vi "Main.vi"(11 "Module Admin":refnum<class "Delacor_lib_QMH_Cloneable Module Admin.lvclass">) -> ()   [LabVIEW 2023, in "TempDataAQuisition.lvlib"]
doc: "This template is based off of the Queued Message Handler design pattern and the Queued Message Handler project template that ships with LabVIEW.\n\nThe main difference is that the queue is private to this module and communication between modules is performed via Broadcast and Request events.\n\nRequest events are wrapped in public API methods and are handled in the Event Handling Loop (EHL) of this VI. Any module can register for Broadcast events sent by this module. The EHL generates messages based on user interface actions.\n\nThe Message Handling Loop (MHL) processes messages generated by the EHL, or by other messages. The messages are string values, so new messages can be added easily to the Message Cases case structure in the MHL. Each message cluster can also provide an optional value for Message Data, which is a variant that can be converted to whatever message-specific data is required.\n_____\nBased on DQMH Project Template 7.0.1.1316."
uses:
  TempDataAQuisition.lvlib
  <vilib>/Delacor/Delacor QMH/Libraries/Cloneable Module Admin_class/Delacor_lib_QMH_Cloneable Module Admin.lvclass
  Module Data--cluster.ctl
  <vilib>/Delacor/Delacor QMH/Libraries/Message Queue_class/Delacor_lib_QMH_Message Queue.lvclass/Delacor_lib_QMH_Message Queue.ctl
  <vilib>/Delacor/Delacor QMH/Libraries/Cloneable Module Admin_class/Delacor_lib_QMH_Cloneable Module Admin.lvclass/Delacor_lib_QMH_Cloneable Module Admin.ctl
  Stop Argument--cluster.ctl
  <vilib>/Delacor/Delacor QMH/Libraries/Module Admin_class/Delacor_lib_QMH_Module Admin.lvclass/Delacor_lib_QMH_Module Admin.ctl
  <vilib>/Utility/miscctls.llb/LVPointTypeDef.ctl
  <vilib>/Delacor/Delacor QMH/Libraries/Message Queue_class/Delacor_lib_QMH_Enqueue Message (Single).vi
  <vilib>/Delacor/Delacor QMH/Libraries/Cloneable Module Admin_class/Delacor_lib_QMH_Get Module ID.vi
  <vilib>/Delacor/Delacor QMH/Libraries/Module Admin_class/Delacor_lib_QMH_Get External Launch.vi
  <vilib>/Delacor/Delacor QMH/Libraries/Message Queue_class/Delacor_lib_QMH_Message Queue.lvclass
  tempRead Argument--cluster.ctl
panel:
  out "error out":errorcluster
  out "Status":string
  in  "Simulate EHL Error":bool
  in  "Simulate MHL Error":bool
  # "Other processes communicate with this Module via its Public API (wrappers for its Request Events).\n\nThis Module communicates with other processes via its Broadcast Events.\nAny process that wants to receive these messages can register for this module's Broadcast events."
  # "This template is for the DQMH framework. See the block diagram for more information on how to use this template."
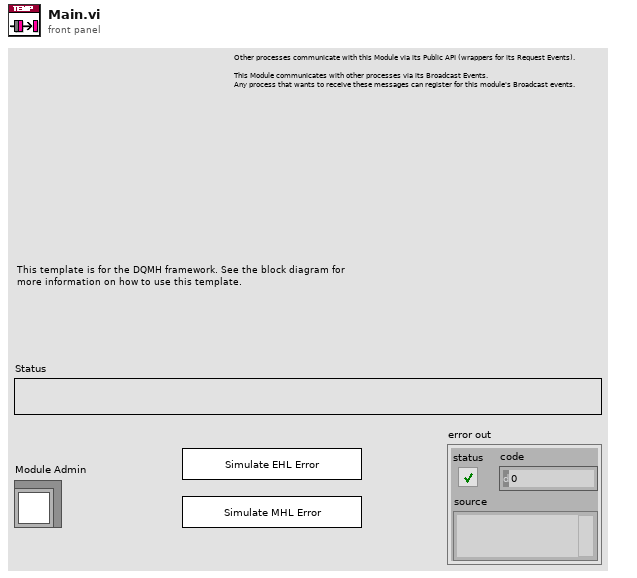
[diagram p1: front panel]
types:
  T1 = typedef "TempDataAQuisition.lvlib/Request Events--cluster.ctl" = cluster{"Stop Module":refnum<user-event>, "Show Panel":refnum<user-event>, "Hide Panel":refnum<user-event>, "Show Diagram":refnum<user-event>, "Get Module Execution Status":refnum<user-event>, "tempRead":refnum<user-event>}
  T2 = typedef "TempDataAQuisition.lvlib/Module Data--cluster.ctl" = cluster{"Status":string}
  T3 = enum32{"invalid lock state", "Not Locked", "Locked (No Password)", "Password-protected"}
  T4 = typedef "TempDataAQuisition.lvlib/Stop Argument--cluster.ctl" = cluster{"Module ID":i32, "Origin":string, "Exit via Stop Module Req?":bool, "Wait for Module to stop?":bool}
  T5 = typedef "TempDataAQuisition.lvlib/tempRead Argument--cluster.ctl" = cluster{"Module ID":i32, "불리언":bool}
  T6 = typedef "LVPointTypeDef.ctl" = cluster{"Horizontal":i16, "Vertical":i16}
  T7 = enum32{"Invalid", "Standard", "Closed", "Hidden", "Minimized", "Maximized"}
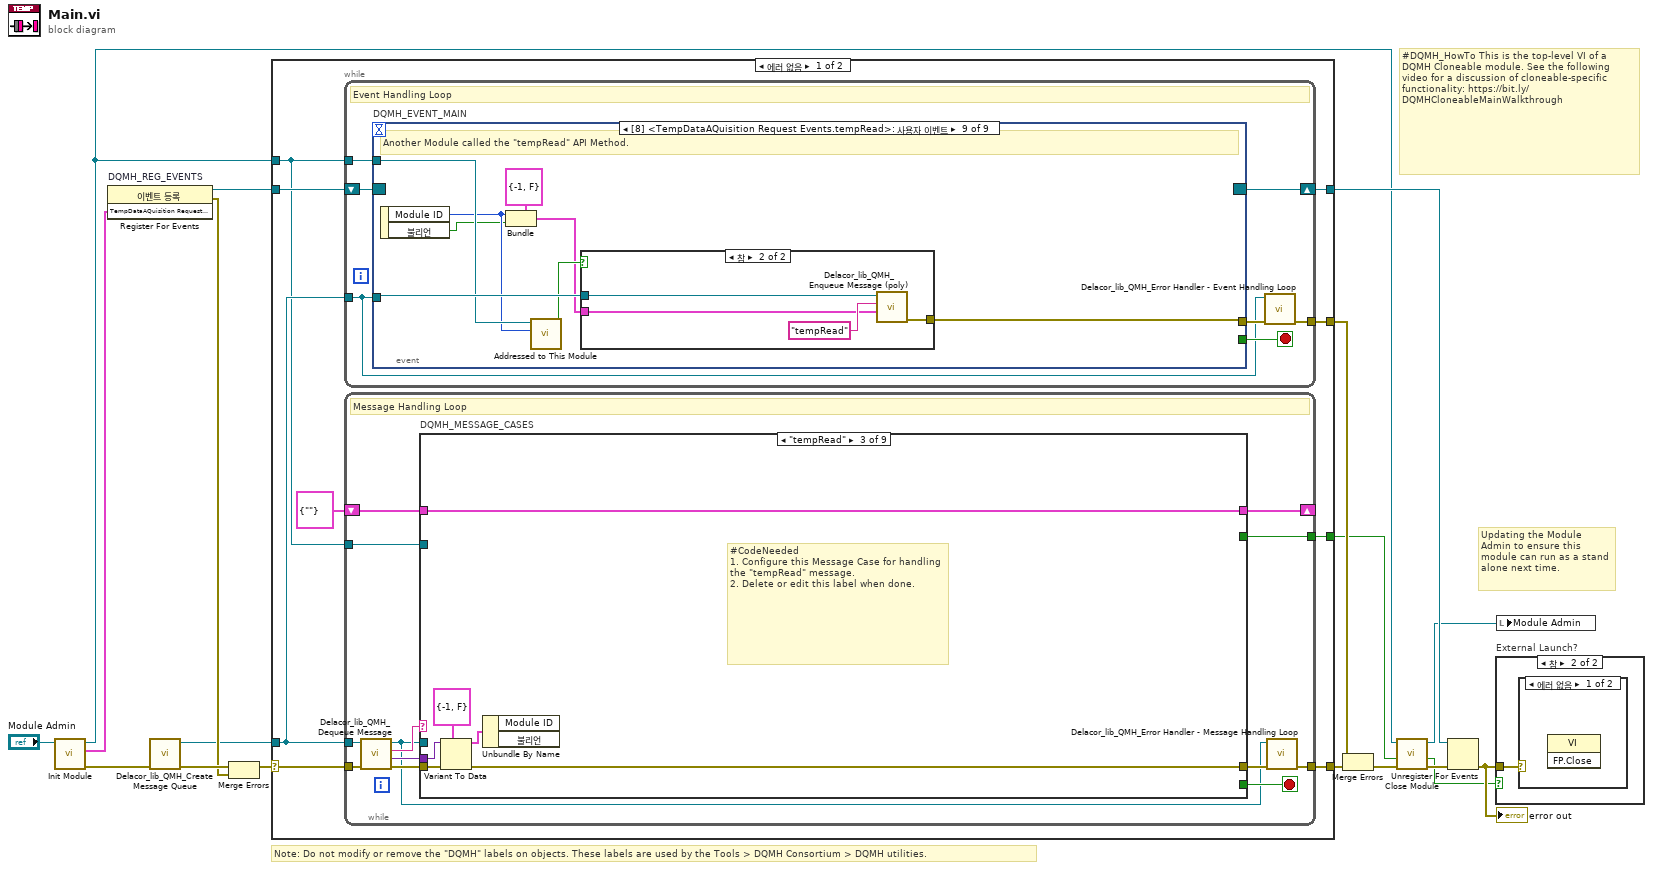
[diagram p0: block diagram]
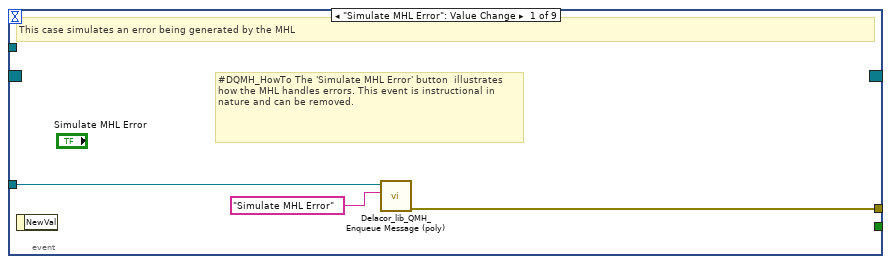
[diagram p2: hidden frame]
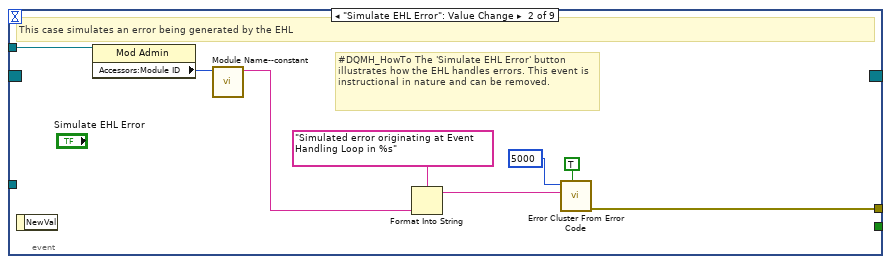
[diagram p3: hidden frame]
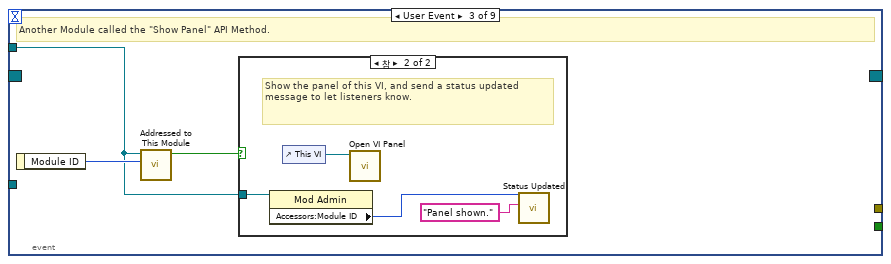
[diagram p4: hidden frame]
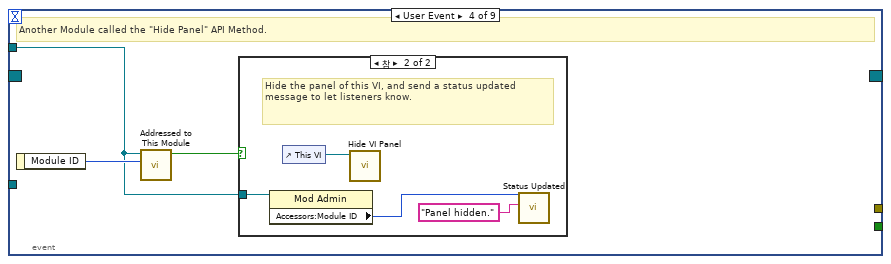
[diagram p6: hidden frame]
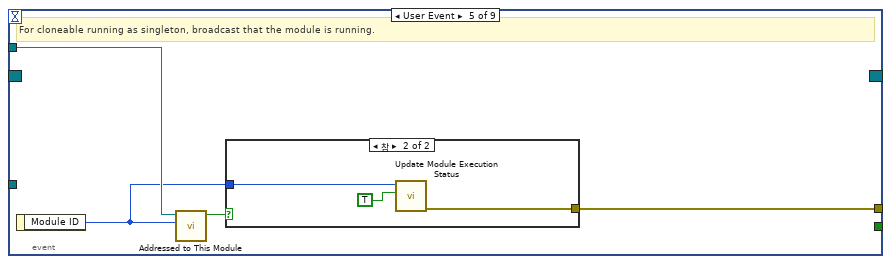
[diagram p8: hidden frame]
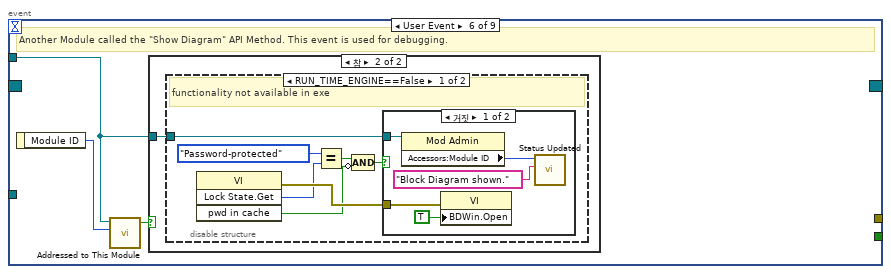
[diagram p10: hidden frame]
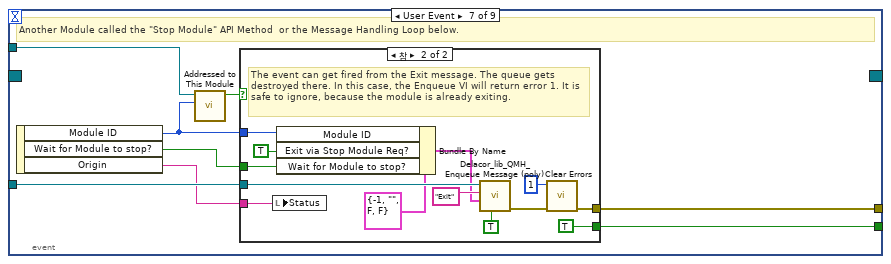
[diagram p14: hidden frame]
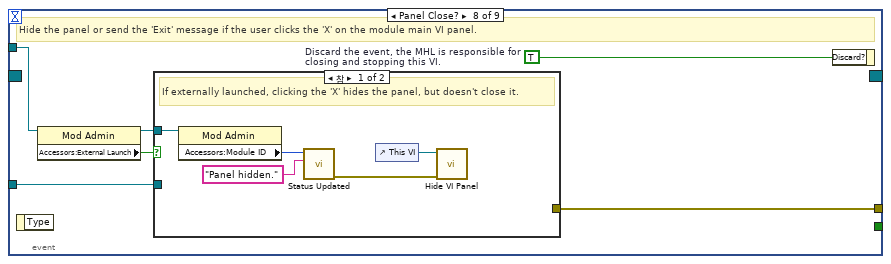
[diagram p16: hidden frame]
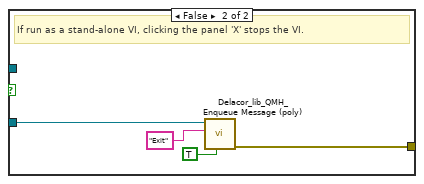
[diagram p17: hidden frame]
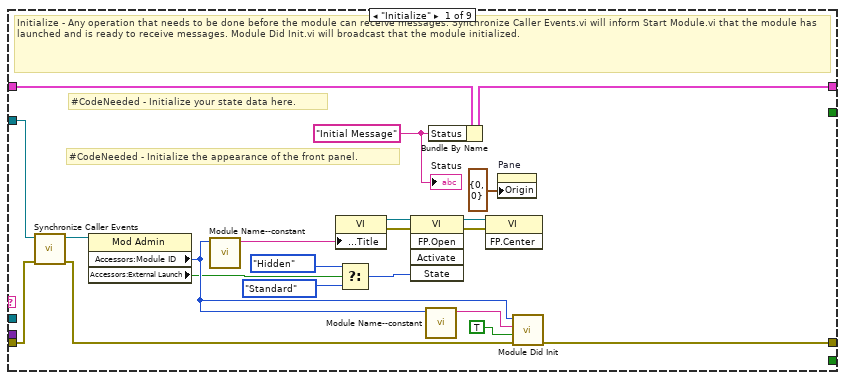
[diagram p19: hidden frame]
diagram:
  # "#DQMH_HowTo This is the top-level VI of a DQMH Cloneable module. See the following video for a discussion of cloneable-specific functionality: https://bit.ly/DQMHCloneableMainWalkthrough"
  # "Note: Do not modify or remove the \"DQMH\" labels on objects. These labels are used by the Tools > DQMH Consortium > DQMH utilities."
  # "Updating the Module Admin to ensure this module can run as a stand alone next time."
  n1 = call "Init Module.vi"("Cloneable Module Admin in"="Module Admin") -> ("error out"=w15:errorcluster, "TempDataAQuisition Request Events"=w7:T1, "Cloneable Module Admin out"=w4:refnum<class "Delacor_lib_QMH_Cloneable Module Admin.lvclass">)  [unwired: 8 in]
  n2 = register-events "DQMH_REG_EVENTS"(w7) -> (reference out=w8:refnum<event-registration>, error out=w10:errorcluster)  [unwired: 2 in]
  n3 = call <vilib>:"Delacor_lib_QMH_Create Message Queue.vi"("error in"=w15) -> ("error out"=w12:errorcluster, "Message Queue"=w6:refnum<class "Delacor_lib_QMH_Message Queue.lvclass">)  [unwired: 9 in]
  n4 = Merge Errors(w12, w10) -> (w11:errorcluster)
  n5 = case shown="에러 없음" w11 {
    selector: w11 -> [w25 w245]
    tunnel: [w27 w244] -> w16
    tunnel: [w24 w243] -> w9
    tunnel: w8 -> [w22 w243]
    tunnel: w6 -> [w21 w236]
    tunnel: [w26 _] -> w17
    tunnel: w4 -> [w20 w239]
    tunnel: [w19 _] -> w2
    frame No Error {
      n6 = while {
        tunnel: w21 -> [w28]
        shift-right: [w31] -> w24
        shift-left: w22 -> [w32]
        tunnel: [w33] -> w26
        tunnel: w20 -> [w29]
        stop <- w30 stop-if-true
        # "Event Handling Loop"
        n7 = event "DQMH_EVENT_MAIN" shown="[8] <TempDataAQuisition Request Events.tempRead>: 사용자 이벤트" {
          selector: w32 -> [_ _ _ _ _ _ _ _ _]
          dyn-events: [_ _ _ _ _ _ _ _ _] -> w31
          timeout: _ -> [_ _ _ _ _ _ _ _ _]
          tunnel: [_ _ _ _ _ _ w86 _ _] -> w30
          tunnel: w28 -> [w36 _ _ _ _ _ w89 w106 w126]
          tunnel: [w37 w45 _ _ w63 _ w90 w109 w119] -> w34
          tunnel: w29 -> [_ w44 w46 w53 w61 w67 w88 w107 w124]
          event "Simulate MHL Error": Value Change {
            # "#DQMH_HowTo The 'Simulate MHL Error' button  illustrates how the MHL handles errors. This event is instructional in nature and can be removed."
            # "This case simulates an error being generated by the MHL"
            n8 = event-data() -> ()  [unwired: 1 in, 1 out]
            n9 = call-poly <vilib>:"Delacor_lib_QMH_Enqueue Message (poly).vi"("Message"="Simulate MHL Error", "Message Queue in"=w36) -> ("error out"=w37:errorcluster)  [unwired: 8 in, 1 out]
          }
          event "Simulate EHL Error": Value Change {
            # "#DQMH_HowTo The 'Simulate EHL Error' button  illustrates how the EHL handles errors. This event is instructional in nature and can be removed."
            # "This case simulates an error being generated by the EHL"
            n10 = event-data() -> ()  [unwired: 1 in, 1 out]
            n11 = property on="Property Node" class="Mod Admin"(reference=w44) -> ("Accessors:Module ID"=w43:i32)  [unwired: 1 in, 2 out]
            n12 = call "Module Name--constant.vi"("Module ID"=w43) -> ("Module Name"=w38:string)  [unwired: 10 in]
            n13 = Format Into String(format string="Simulated error originating at Event Handling Loop in %s", w38) -> (resulting string=w41:string)  [unwired: 2 in, 1 out]
            n14 = call <vilib>:"Error Cluster From Error Code.vi"("show call chain? (False)"=TRUE, "error message (\"\")"=w41, "error code (0)"=5000) -> ("error out"=w45:errorcluster)  [unwired: 6 in]
          }
          event User Event {
            # "Another Module called the \"Show Panel\" API Method."
            n15 = event-data() -> ("Module ID"=w47:i32)  [unwired: 1 in]
            n16 = call "Addressed to This Module.vi"("Module ID from Argument"=w47, "Module Admin"=w46) -> ("Addressed to this instance?"=w48:bool)  [unwired: 8 in, 1 out]
            n17 = case shown="참" w48 {
              tunnel: w46 -> [_ w50]
              frame False {
              }
              frame True {
                # "Show the panel of this VI, and send a status updated message to let listeners know."
                n18 = property on="Property Node" class="Mod Admin"(reference=w50) -> ("Accessors:Module ID"=w49:i32)  [unwired: 1 in, 2 out]
                n19 = control-ref of="This VI"() -> (w52:refnum<vi>)
                n20 = call "Open VI Panel.vi"("VI"=w52) -> ()  [unwired: 10 in, 1 out]
                n21 = call "Status Updated.vi"("Status"="Panel shown." ("format string"), "Module ID"=w49) -> ()  [unwired: 9 in, 1 out]
              }
            }
          }
          event User Event {
            # "Another Module called the \"Hide Panel\" API Method."
            n22 = event-data() -> ("Module ID"=w54:i32)  [unwired: 1 in]
            n23 = call "Addressed to This Module.vi"("Module ID from Argument"=w54, "Module Admin"=w53) -> ("Addressed to this instance?"=w55:bool)  [unwired: 8 in, 1 out]
            n24 = case shown="참" w55 {
              tunnel: w53 -> [_ w57]
              frame False {
              }
              frame True {
                # "Hide the panel of this VI, and send a status updated message to let listeners know."
                n25 = property on="Property Node" class="Mod Admin"(reference=w57) -> ("Accessors:Module ID"=w56:i32)  [unwired: 1 in, 2 out]
                n26 = control-ref of="This VI"() -> (w59:refnum<vi>)
                n27 = call "Hide VI Panel.vi"("VI"=w59) -> ()  [unwired: 10 in, 1 out]
                n28 = call "Status Updated.vi"("Status"="Panel hidden." ("format string"), "Module ID"=w56) -> ()  [unwired: 9 in, 1 out]
              }
            }
          }
          event User Event {
            # "For cloneable running as singleton, broadcast that the module is running."
            n29 = event-data() -> ("Module ID"=w60:i32)  [unwired: 1 in]
            n30 = call "Addressed to This Module.vi"("Module ID from Argument"=w60, "Module Admin"=w61) -> ("Addressed to this instance?"=w62:bool)  [unwired: 8 in, 1 out]
            n31 = case shown="참" w62 {
              tunnel: [_ w66] -> w63
              tunnel: w60 -> [_ w65]
              frame False {
              }
              frame True {
                n32 = call "Update Module Execution Status.vi"("Running?"=TRUE, "Module ID"=w65) -> ("error out"=w66:errorcluster)  [unwired: 9 in]
              }
            }
          }
          event User Event {
            # "Another Module called the \"Show Diagram\" API Method. This event is used for debugging."
            n33 = event-data() -> ("Module ID"=w68:i32)  [unwired: 1 in]
            n34 = call "Addressed to This Module.vi"("Module ID from Argument"=w68, "Module Admin"=w67) -> ("Addressed to this instance?"=w69:bool)  [unwired: 8 in, 1 out]
            n35 = case shown="참" w69 {
              tunnel: w67 -> [_ w70]
              frame False {
              }
              frame True {
                n36 = disable-structure shown="RUN_TIME_ENGINE==False" {
                  disable-tunnel: w70 -> [w71 _]
                  frame condition #0 (active) {
                    # "functionality not available in exe"
                    n37 = invoke on="Invoke Node" class="VI" method="Lock State.Get"() -> (error out=w77:errorcluster, "Get Lock State"=w76:T3, "pwd in cache"=w73:bool)  [unwired: 4 in, 1 out]
                    n38 = Equal?(x=T3."Password-protected", y=w76) -> (x = y?=w74:bool)
                    n39 = Compound Arithmetic op=AND(w74, invert w73) -> (w72:bool)
                    n40 = case shown="거짓" w72 {
                      tunnel: w77 -> [w82 _]
                      tunnel: w71 -> [w79 _]
                      frame False {
                        n41 = property on="Property Node" class="Mod Admin"(reference=w79) -> ("Accessors:Module ID"=w78:i32)  [unwired: 1 in, 2 out]
                        n42 = property on="Property Node" class="VI"(error in=w82, "BDWin.Open"=TRUE ("Block Diagram Window:Open")) -> ()  [unwired: 1 in, 2 out]
                        n43 = call "Status Updated.vi"("Status"="Block Diagram shown." ("format string"), "Module ID"=w78) -> ()  [unwired: 9 in, 1 out]
                      }
                      frame True {
                        # "Password-protected VI, and the password is not in the cache. Do not show the diagram."
                      }
                    }
                  }
                  frame condition #1 {
                  }
                }
              }
            }
          }
          event User Event {
            # "Another Module called the \"Stop Module\" API Method  or the Message Handling Loop below."
            n44 = event-data() -> ("Module ID"=w84:i32, "Wait for Module to stop?"=w85:bool, "Origin"=w83:string)  [unwired: 1 in]
            n45 = call "Addressed to This Module.vi"("Module ID from Argument"=w84, "Module Admin"=w88) -> ("Addressed to this instance?"=w87:bool)  [unwired: 8 in, 1 out]
            n46 = case shown="참" w87 {
              tunnel: [_ w102] -> w90
              tunnel: w89 -> [_ w98]
              tunnel: [_ TRUE] -> w86
              tunnel: w85 -> [_ w93]
              tunnel: w84 -> [_ w95]
              tunnel: w83 -> [_ w91]
              frame False {
              }
              frame True {
                # "The event can get fired from the Exit message. The queue gets destroyed there. In this case, the Enqueue VI will return error 1. It is safe to ignore, because the module is already exiting."
                n47 = local write "Status"(w91) -> ()
                n48 = Bundle By Name(cluster=T4 {"Module ID"=-1, "Origin"="", "Exit via Stop Module Req?"=FALSE, "Wait for Module to stop?"=FALSE} ("Stop Argument"), "Module ID"=w95, "Exit via Stop Module Req?"=TRUE, "Wait for Module to stop?"=w93) -> (w92:T4)
                n49 = call-poly <vilib>:"Delacor_lib_QMH_Enqueue Message (poly).vi"("Priority Message? (F)"=TRUE, "Message Data"=w92, "Message"="Exit", "Message Queue in"=w98) -> ("error out"=w103:errorcluster)  [unwired: 6 in, 1 out]
                n50 = call <vilib>:"Clear Errors.vi"("error in (no error)"=w103, "specific error code to clear (0: all)"=1) -> ("error out"=w102:errorcluster)  [unwired: 4 in, 1 out]
              }
            }
          }
          event Panel Close? {
            w108 = TRUE  # Discard the event, the MHL is responsible for closing and stopping this VI.
            # "Hide the panel or send the 'Exit' message if the user clicks the 'X' on the module main VI panel."
            n51 = event-data() -> ()  [unwired: 1 in, 1 out]
            n52 = property on="Property Node" class="Mod Admin"(reference=w107) -> (reference out=w104:refnum<class "Delacor_lib_QMH_Cloneable Module Admin.lvclass">, "Accessors:External Launch"=w105:bool)  [unwired: 1 in, 1 out]
            n53 = case shown="참" w105 {
              tunnel: w106 -> [_ w117]
              tunnel: [_ w118] -> w109
              tunnel: w104 -> [w112 _]
              frame True {
                # "If externally launched, clicking the 'X' hides the panel, but doesn't close it."
                n54 = property on="Property Node" class="Mod Admin"(reference=w112) -> ("Accessors:Module ID"=w111:i32)  [unwired: 1 in, 2 out]
                n55 = call "Status Updated.vi"("Status"="Panel hidden." ("format string"), "Module ID"=w111) -> ("error out"=w110:errorcluster)  [unwired: 9 in]
                n56 = control-ref of="This VI"() -> (w114:refnum<vi>)
                n57 = call "Hide VI Panel.vi"("error in"=w110, "VI"=w114) -> ()  [unwired: 9 in, 1 out]
              }
              frame False {
                # "If run as a stand-alone VI, clicking the panel 'X' stops the VI."
                n58 = call-poly <vilib>:"Delacor_lib_QMH_Enqueue Message (poly).vi"("Priority Message? (F)"=TRUE, "Message"="Exit", "Message Queue in"=w117) -> ("error out"=w118:errorcluster)  [unwired: 7 in, 1 out]
              }
            }
            n59 = event-data ("Event Filter Node")("Discard?"=w108) -> ()  [unwired: 1 in, 1 out]
          }
          event User Event {
            # "Another Module called the \"tempRead\" API Method."
            n60 = event-data() -> ("Module ID"=w121:i32, "불리언"=w120:bool)  [unwired: 1 in]
            n61 = Bundle(cluster=T5 {"Module ID"=-1, "불리언"=FALSE} ("tempRead Argument"), "Module ID"=w121, "불리언"=w120) -> (w122:T5)
            n62 = call "Addressed to This Module.vi"("Module ID from Argument"=w121, "Module Admin"=w124) -> ("Addressed to this instance?"=w125:bool)  [unwired: 8 in, 1 out]
            n63 = case "케이스 구조" shown="참" w125 {
              tunnel: w126 -> [_ w130]
              tunnel: w122 -> [_ w128]
              tunnel: [_ w127] -> w119
              frame False {
              }
              frame True {
                n64 = call-poly <vilib>:"Delacor_lib_QMH_Enqueue Message (poly).vi"("Message Data"=w128, "Message"="tempRead", "Message Queue in"=w130) -> ("error out"=w127:errorcluster)  [unwired: 7 in, 1 out]
              }
            }
          }
        }
        n65 = call-dynamic "Delacor_lib_QMH_Error Handler - Event Handling Loop.vi"("error in"=w34, "Message Queue in"=w28) -> ("dup error in"=w33:errorcluster)  [unwired: 8 in, 1 out]
      }
      n66 = while {
        tunnel: w21 -> [w131]
        shift-right: [w138] -> _
        shift-left: T2 {"Status"=""} ("Data Cluster") -> [w139]
        tunnel: w25 -> [w142]
        tunnel: [w140] -> w27
        tunnel: w20 -> [w133]
        tunnel: [w132] -> w19
        stop <- w137 stop-if-true
        # "Message Handling Loop"
        n67 = call-dynamic "Delacor_lib_QMH_Dequeue Message.vi"("error in"=w142, "Message Queue in"=w131) -> ("error out"=w141:errorcluster, "Message Data"=w135:variant, "Message"=w136:string, "Message Queue out"=w134:refnum<class "Delacor_lib_QMH_Message Queue.lvclass">)  [unwired: 6 in]
        n68 = case "DQMH_MESSAGE_CASES" shown="\"tempRead\"" w136 {
          selector: w136 -> [_ _ _ _ _ _ _ _ w225]
          tunnel: w134 -> [_ _ _ _ _ w180 _ w217 _]
          tunnel: w141 -> [w162 w166 w172 w175 w177 w189 w206 w223 w234]
          tunnel: [w160 w166 w170 w174 w177 w185 w205 w218 w235] -> w143
          tunnel: w139 -> [w153 w165 w171 w173 w176 w184 w203 w216 w232]
          tunnel: [w152 w165 w171 w173 w176 w184 w203 w216 w232] -> w138
          tunnel: [_ _ _ _ _ _ _ w215 _] -> w137
          tunnel: w135 -> [_ _ w169 _ _ w183 _ w213 _]
          tunnel: w133 -> [w147 _ _ _ _ w182 w201 w208 w231]
          tunnel: [_ _ _ _ _ _ _ w211 _] -> w132
          frame "Initialize" {
            w144 = "Initial Message" ("Initial Message")
            # "#CodeNeeded - Initialize the appearance of the front panel."
            # "#CodeNeeded - Initialize your state data here."
            # "Initialize - Any operation that needs to be done before the module can receive messages. Synchronize Caller Events.vi will inform Start Module.vi that the module has launched and is ready to receive messages. Module Did Init.vi will broadcast that the module initialized."
            n69 = call "Synchronize Caller Events.vi"("error in"=w162, "Module Admin"=w147) -> ("error out"=w161:errorcluster, "Module Admin out"=w146:refnum<class "Delacor_lib_QMH_Cloneable Module Admin.lvclass">)  [unwired: 8 in]
            n70 = property on="Property Node" class="Mod Admin"(reference=w146) -> ("Accessors:Module ID"=w149:i32, "Accessors:External Launch"=w148:bool)  [unwired: 1 in, 2 out]
            n71 = call "Module Name--constant.vi"("Module ID"=w149) -> ("Module Name"=w157:string)  [unwired: 10 in]
            n72 = property on="Property Node" class="VI"("Front Panel.Title"=w157) -> (reference out=w159:refnum<vi>, error out=w164:errorcluster)  [unwired: 2 in]
            n73 = Select(t=T7."Hidden" ("State"), s=w148, f=T7."Standard" ("State")) -> (s? t:f=w154:T7)
            n74 = invoke on="Invoke Node" class="VI" method="FP.Open"(reference=w159, error in=w164, "State"=w154) -> (reference out=w158:refnum<vi>, error out=w163:errorcluster)  [unwired: 2 in, 3 out]
            n75 = call "Module Name--constant.vi"("Module ID"=w149) -> ("Module Name"=w150:string)  [unwired: 10 in]
            n76 = Bundle By Name(cluster=w153, "Status"=w144) -> (w152:T2)
            n77 = invoke on="Invoke Node" class="VI" method="FP.Center"(reference=w158, error in=w163) -> ()  [unwired: 1 in, 3 out]
            n78 = property on="Pane" class="Pane"("Origin"=T6 {"Horizontal"=0, "Vertical"=0}) -> ()  [unwired: 2 in, 2 out]
            n79 = call "Module Did Init.vi"("error in"=w161, "Initialized?"=TRUE, "Origin"=w150, "Module ID"=w149) -> ("error out"=w160:errorcluster)  [unwired: 7 in]
            "Status" <- w144
          }
          frame "---Module Specific---" {
            # "Separator -- The following cases handle messages specific to this Module."
          }
          frame "tempRead" {
            # "#CodeNeeded\n1. Configure this Message Case for handling the \"tempRead\" message.\n2. Delete or edit this label when done."
            n80 = Variant To Data(error in=w172, type=T5 {"Module ID"=-1, "불리언"=FALSE} ("tempRead Argument"), Variant=w169) -> (data=w167:T5, error out=w170:errorcluster)
            n81 = Unbundle By Name(w167) -> ()  [unwired: 2 out]
          }
          frame "---Copy This Frame---" {
            # "Duplicate this frame when creating new messages.  Change this comment in the duplicated frame to describe this message."
            n82 = Merge Errors(w175) -> (w174:errorcluster)
          }
          frame "---Exit and Error Handling---" {
            # "Separator - the following cases handle errors and exit messages."
          }
          frame "Error" {
            # "#CodeRecommended - If the module is running in standalone mode (External Launch = FALSE), this code will pop up an error dialog and call the 'Exit' message if an error occurs. Add more fine-grained error management here."
            # "Error - Check the error message data and respond accordingly. This message is sent by the \"Error Handler\" VIs at the end of each loop in this application."
            n83 = property on="Property Node" class="Mod Admin"(reference=w182) -> ("Accessors:External Launch"=w181:bool, "Accessors:Module ID"=w179:i32)  [unwired: 1 in, 2 out]
            n84 = Variant To Data(error in=w189, type=errorcluster {"status"=FALSE, "code"=0, "source"=""} ("error constant"), Variant=w183) -> (data=w178:errorcluster, error out=w187:errorcluster)
            n85 = local write "error out"(w178) -> ()
            n86 = call "Error Reported.vi"("Error"=w178, "Module ID"=w179) -> ()  [unwired: 9 in, 1 out]
            n87 = case shown="거짓" w181 {
              tunnel: [w194 _] -> w186
              tunnel: w180 -> [w192 _]
              tunnel: w178 -> [w193 _]
              frame False {
                n88 = disable-structure shown="DQMH_Disable_SEH==TRUE" {
                  disable-tunnel: w193 -> [w195 _]
                  frame condition #0 (active) {
                    # "If the module is running standalone, then pop up an error dialog and call the \"Exit\" message."
                    n89 = call <vilib>:"Simple Error Handler.vi"("error in (no error)"=w195) -> ()  [unwired: 4 in, 5 out]
                  }
                  frame condition #1 {
                    # "To prevent the Simple Error Handler VI from being loaded (e.g. when deploying to a Real-Time target), add the Conditional Disable Symbol \"DQMH_Disable_SEH\" to your project and set it to TRUE."
                  }
                }
                n90 = call-poly <vilib>:"Delacor_lib_QMH_Enqueue Message (poly).vi"("Priority Message? (F)"=TRUE, "Message"="Exit", "Message Queue in"=w192) -> ("error out"=w194:errorcluster)  [unwired: 7 in, 1 out]
              }
              frame True {
                # "If the module was launched externally, calling the Error Reported broadcast VI is the only action performed by the \"Error\" message. The module's caller can then process the error appropriately."
              }
            }
            n91 = Merge Errors(w187, w186) -> (w185:errorcluster)
          }
          frame "Simulate MHL Error" {
            # "#DQMH_HowTo The 'Simulate MHL Error' button  illustrates how the MHL handles errors. This event is instructional in nature and can be removed."
            # "Simulate an error occurring at the MHL"
            n92 = property on="Property Node" class="Mod Admin"(reference=w201) -> ("Accessors:Module ID"=w202:i32)  [unwired: 1 in, 2 out]
            n93 = call "Module Name--constant.vi"("Module ID"=w202) -> ("Module Name"=w197:string)  [unwired: 10 in]
            n94 = Format Into String(format string="Simulated error originating at Message Handling Loop in %s", w197) -> (resulting string=w198:string)  [unwired: 2 in, 1 out]
            n95 = call <vilib>:"Error Cluster From Error Code.vi"("show call chain? (False)"=TRUE, "error message (\"\")"=w198, "error code (0)"=5001) -> ("error out"=w204:errorcluster)  [unwired: 6 in]
            n96 = Merge Errors(w206, w204) -> (w205:errorcluster)
          }
          frame "Exit" {
            w214 = 91  # 91: not all Exit messages will have an argument
            w215 = TRUE  # Stop the VI
            # "Release the message queue reference"
            # "#CodeNeeded - Add any required cleanup code here."
            # "Exit - Exit the application."
            n97 = Variant To Data(error in=w223, type=T4 {"Module ID"=-1, "Origin"="", "Exit via Stop Module Req?"=FALSE, "Wait for Module to stop?"=FALSE} ("Stop Argument"), Variant=w213) -> (data=w210:T4, error out=w219:errorcluster)
            n98 = call <vilib>:"Clear Errors.vi"("error in (no error)"=w219, "specific error code to clear (0: all)"=w214) -> ("error out"=w222:errorcluster)  [unwired: 4 in, 1 out]
            n99 = property on="Property Node" class="Mod Admin"(reference=w208) -> ("Accessors:Module ID"=w207:i32)  [unwired: 1 in, 2 out]
            n100 = control-ref of="This VI"() -> (w209:refnum<vi>)
            n101 = call-dynamic "Delacor_lib_QMH_Release Message Queue.vi"("error in"=w222, "Message Queue"=w217) -> ("error out"=w221:errorcluster)  [unwired: 9 in]
            n102 = call "Handle Exit.vi"("Stop Argument"=w210, "Module Admin in"=w208, "VI reference"=w209) -> ("error out"=w220:errorcluster, "Wait for Stop?"=w211:bool)  [unwired: 7 in]
            n103 = Merge Errors(w221, w220) -> (w218:errorcluster)
            n104 = call "Error Reported.vi"("Error"=w218, "Module ID"=w207) -> ()  [unwired: 9 in, 1 out]
          }
          frame Default {
            # "'Default' case only runs if there is a message that isn't defined in any of the other cases.  Output a programming error."
            n105 = property on="Property Node" class="Mod Admin"(reference=w231) -> ("Accessors:Module ID"=w230:i32)  [unwired: 1 in, 2 out]
            n106 = call "Module Name--constant.vi"("Module ID"=w230) -> ("Module Name"=w224:string)  [unwired: 10 in]
            n107 = Format Into String(format string="The invalid message string \"%s\" was received in the Message Handling Loop for module \"%s\".", w225, w224) -> (resulting string=w227:string)  [unwired: 2 in, 1 out]
            n108 = call <vilib>:"Error Cluster From Error Code.vi"("show call chain? (False)"=TRUE, "error message (\"\")"=w227, "error code (0)"=1) -> ("error out"=w233:errorcluster)  [unwired: 6 in]
            n109 = Merge Errors(w234, w233) -> (w235:errorcluster)
          }
        }
        n110 = call-dynamic "Delacor_lib_QMH_Error Handler - Message Handling Loop.vi"("error in"=w143, "Message Queue in"=w134) -> ("dup error in"=w140:errorcluster)  [unwired: 8 in, 1 out]
      }
    }
    frame Error {
      n111 = call "Synchronize Caller Events.vi"("Module Admin"=w239) -> ("Module Admin out"=w238:refnum<class "Delacor_lib_QMH_Cloneable Module Admin.lvclass">)  [unwired: 9 in, 1 out]
      n112 = property on="Property Node" class="Mod Admin"(reference=w238) -> ("Accessors:Module ID"=w237:i32)  [unwired: 1 in, 2 out]
      n113 = call-dynamic "Delacor_lib_QMH_Release Message Queue.vi"("error in"=w245, "Message Queue"=w236) -> ("error out"=w244:errorcluster)  [unwired: 9 in]
      n114 = call "Module Name--constant.vi"("Module ID"=w237) -> ("Module Name"=w242:string)  [unwired: 10 in]
      n115 = Format Into String(format string="An error occurred during initialization. %s is no longer running.", w242) -> (resulting string=w240:string)  [unwired: 2 in, 1 out]
      n116 = call "Error Reported.vi"("Additional Information"=w240, "Error"=w244, "Module ID"=w237) -> ()  [unwired: 8 in, 1 out]
    }
  }
  n117 = Merge Errors(w17, w16) -> (w18:errorcluster)
  n118 = call "Close Module.vi"("error in"=w18, "Wait for stop?"=w2, "Module Admin in"=w4) -> ("error out"=w14:errorcluster, "External Launch"=w1:bool, "Module Admin out"=w3:refnum<class "Delacor_lib_QMH_Cloneable Module Admin.lvclass">)  [unwired: 6 in]
  n119 = Unregister For Events(event registration refnum=w9, error in=w14) -> (error out=w13:errorcluster)
  "error out" <- w13
  n120 = case "External Launch?" shown="참" w1 {
    tunnel: w13 -> [_ w246]
    frame False {
    }
    frame True {
      n121 = case shown="에러 없음" w246 {
        frame No Error {
          n122 = invoke class="VI" method="FP.Close"() -> ()  [unwired: 3 in, 3 out]
        }
        frame Error {
          n123 = invoke class="VI" method="FP.Open"("Activate"=TRUE ("Activate?")) -> ()  [unwired: 4 in, 5 out]
        }
      }
    }
  }
  n124 = local write "Module Admin"(w3) -> ()
